vi "Write Lockin Processor Configuration.vi"(8 "error in (no error)":errorcluster, 10 "Configuration":T1={"Time constant"=0.0, "Signal channels"=[], "Group"="p", "X channel"="", "Live update"=TRUE, "Phases"=[], "Harmonics"=[]} {"Phases" scale=-180.0..180.0; "Time constant" min=1e-06 max=1.0 scale=1e-06..0.01 scale format="%#_6p"}, 11 "Lockin Processor in":refnum<class "Lockin Processor.lvclass">) -> (0 "error out":errorcluster, 3 "Lockin Processor out":refnum<class "Lockin Processor.lvclass">)   [LabVIEW 2016, in "Lockin Processor.lvclass"]
uses:
  Lockin Processor.lvclass
  C:/github/LabActor/Template Module/Template Module.lvclass
  Lockin Processor Configuration.ctl
  Template Module/Template Module.lvclass/Template Module.ctl
  Template Module/Write Configuration.vi
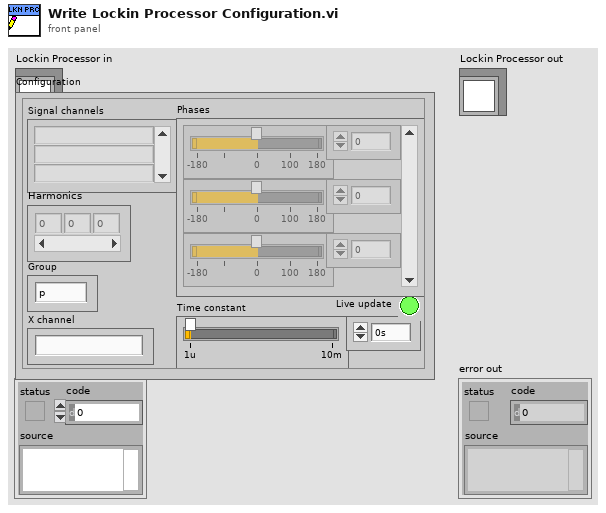
[diagram p1: front panel]
types:
  T1 = typedef "Lockin Processor Configuration.ctl" = cluster{"Time constant":dbl, "Signal channels":string[], "Group":string, "X channel":string, "Live update":bool, "Phases":dbl[], "Harmonics":i32[]}
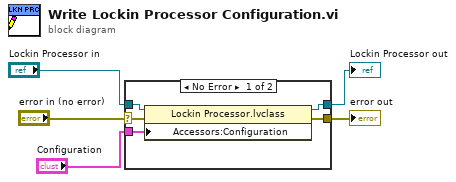
[diagram p0: block diagram]
diagram:
  n1 = case shown="No Error" "error in (no error)" {
    selector: "error in (no error)" -> [w8 w11]
    tunnel: [w6 w11] -> w4
    tunnel: [w7 w12] -> w2
    tunnel: "Lockin Processor in" -> [w10 w12]
    tunnel: "Configuration" -> [w9 _]
    frame No Error {
      n2 = property class="Lockin Processor.lvclass"(reference=w10, error in=w8, "Accessors:Configuration"=w9) -> (reference out=w7:refnum<class "Lockin Processor.lvclass">, error out=w6:errorcluster)
    }
    frame Error {
    }
  }
  "error out" <- w4
  "Lockin Processor out" <- w2
